vi "HFRR ADV v013 new software.vi"() -> ()   [LabVIEW 2025] (continued)
      event "Calibration": Value Change {
        n342 = event-data() -> ()  [unwired: 1 in, 6 out]
        n343 = local read "Calibration"() -> (w428:bool)
        n344 = case shown="False" w428 {
          frame False {
            n345 = property on="Calibration 2" class="TabCtl (strict)"("Visible"=FALSE) -> ()  [unwired: 2 in, 2 out]
            n346 = local write "Cal Password"("" ("Cal Password")) -> ()
          }
          frame True {
            n347 = property on="Calibration 2" class="TabCtl (strict)"("Visible"=TRUE) -> ()  [unwired: 2 in, 2 out]
            n348 = local write "Cal Password"("" ("Cal Password")) -> ()
          }
        }
        n349 = property on="Wrong Password" class="Str"("Visible"=FALSE) -> ()  [unwired: 2 in, 2 out]
      }
      event "Cal Password": Value Change {
        n350 = event-data() -> ()  [unwired: 1 in, 6 out]
        n351 = local read "Cal Password"() -> (w436:string)
        n352 = call <vilib>:"Trim Whitespace.vi"("string"=w436) -> ("trimmed string"=w435:string)  [unwired: 1 in]
        n353 = Equal?(x=w435, y="Cal@321") -> (x = y?=w433:bool)
        n354 = case shown="True" w433 {
          frame False {
            n355 = property on="Wrong Password" class="Str"("Visible"=TRUE) -> ()  [unwired: 2 in, 2 out]
          }
          frame True {
            n356 = property on="Wrong Password" class="Str"("Visible"=FALSE) -> ()  [unwired: 2 in, 2 out]
            n357 = local write "Main Tab"(T2."About" ("Main Tab")) -> ()
            n358 = local write "Cal Password"("" ("Cal Password")) -> ()
            n359 = local write "Main Dashboard Buttons"(T1."About" ("Main Dashboard Buttons")) -> ()
            n360 = local write "Tab Control 5"(T11."Temperature Calibration" ("Tab Control 5")) -> ()
            n361 = property on="Calibration 2" class="TabCtl (strict)"("Visible"=FALSE) -> ()  [unwired: 2 in, 2 out]
            n362 = property on="Tab Control 5" class="TabCtl (strict)"("Tabs Visible?"=FALSE ("Page Labels Display Visible?")) -> ()  [unwired: 2 in, 2 out]
            n363 = local write "Calibration"(FALSE ("Calibration")) -> ()
          }
        }
      }
      event "Calibration Selection": Value Change {
        n364 = event-data() -> ()  [unwired: 1 in, 6 out]
        n365 = local read "Calibration Selection"() -> (w447:T8)
        n366 = case shown="\"Stroke Calibration\"" w447 {
          tunnel: [T7."Stroke" ("Main Calibration Tab") T7."Friction" ("Main Calibration Tab") T7."Main" ("Main Calibration Tab") T7."Temperature" ("Main Calibration Tab")] -> w446
          frame "Stroke Calibration" {
          }
          frame "Friction Force Calibration" {
          }
          frame Default {
          }
          frame "Temperature Calibration" {
          }
        }
        n367 = local write "Main Calibration Tab"(w446) -> ()
      }
      event "Back Stroke": Value Change {
        n368 = event-data() -> ()  [unwired: 1 in, 6 out]
        n369 = local write "Main Stroke Tab"(T9."Step 1" ("Main Stroke Tab")) -> ()
        n370 = local write "Main Calibration Tab"(T7."Main" ("Main Calibration Tab")) -> ()
        n371 = local write "Back Stroke"(FALSE ("Back Stroke")) -> ()
      }
      event "Step 2 Back": Value Change {
        n372 = event-data() -> ()  [unwired: 1 in, 6 out]
        n373 = local write "Main Stroke Tab"(T9."Step 1" ("Main Stroke Tab")) -> ()
        n374 = local write "Step 2 Back"(FALSE ("Back Stroke")) -> ()
      }
      event "Step 3 Back": Value Change {
        n375 = event-data() -> ()  [unwired: 1 in, 6 out]
        n376 = local write "Main Stroke Tab"(T9."Step 2" ("Main Stroke Tab")) -> ()
        n377 = local write "Step 3 Back"(FALSE ("Back Stroke")) -> ()
      }
      event "Step 4 Back": Value Change {
        n378 = event-data() -> ()  [unwired: 1 in, 6 out]
        n379 = local write "Main Stroke Tab"(T9."Step 3" ("Main Stroke Tab")) -> ()
        n380 = local write "Step 4 Back"(FALSE ("Back Stroke")) -> ()
      }
      event "Step 5 Back": Value Change {
        n381 = event-data() -> ()  [unwired: 1 in, 6 out]
        n382 = local write "Main Stroke Tab"(T9."Step 4" ("Main Stroke Tab")) -> ()
        n383 = local write "Step 5 Back"(FALSE ("Back Stroke")) -> ()
      }
      event "Step 6 Back": Value Change {
        n384 = event-data() -> ()  [unwired: 1 in, 6 out]
        n385 = local write "Main Stroke Tab"(T9."Step 5" ("Main Stroke Tab")) -> ()
        n386 = local write "Step 6 Back"(FALSE ("Back Stroke")) -> ()
      }
      event "Back Stroke step 7": Value Change {
        n387 = event-data() -> ()  [unwired: 1 in, 6 out]
        n388 = local write "Main Stroke Tab"(T9."Step 6" ("Main Stroke Tab")) -> ()
        n389 = local write "Back Stroke step 7"(FALSE ("Back Stroke")) -> ()
      }
      event "Back Stroke step 8": Value Change {
        n390 = event-data() -> ()  [unwired: 1 in, 6 out]
        n391 = local write "Main Stroke Tab"(T9."Step 7" ("Main Stroke Tab")) -> ()
        n392 = local write "Back Stroke step 8"(FALSE ("Back Stroke")) -> ()
      }
      event "Back Stroke 8": Value Change {
        n393 = event-data() -> ()  [unwired: 1 in, 6 out]
        n394 = local write "MOVE CARRIAGE TO"(0.0 ("MOVE CARRIAGE TO")) -> ()
        n395 = local write "Main Stroke Tab"(T9."Step 1" ("Main Stroke Tab")) -> ()
        n396 = local write "Back Stroke 8"(FALSE ("Back Stroke 8")) -> ()
      }
      event "Continue Stroke": Value Change {
        n397 = event-data() -> ()  [unwired: 1 in, 6 out]
        n398 = local write "Main Stroke Tab"(T9."Step 2" ("Main Stroke Tab")) -> ()
        n399 = local write "Continue Stroke"(FALSE ("Continue Stroke")) -> ()
      }
      event "Continue Stroke step 2": Value Change {
        n400 = event-data() -> ()  [unwired: 1 in, 6 out]
        n401 = local write "Main Stroke Tab"(T9."Step 3" ("Main Stroke Tab")) -> ()
        n402 = local write "Continue Stroke step 2"(FALSE ("Continue Stroke")) -> ()
      }
      event "Continue Stroke step 3": Value Change {
        n403 = event-data() -> ()  [unwired: 1 in, 6 out]
        n404 = local write "Main Stroke Tab"(T9."Step 4" ("Main Stroke Tab")) -> ()
        n405 = local write "Continue Stroke step 3"(FALSE ("Continue Stroke")) -> ()
      }
      event "Continue Stroke step 4": Value Change {
        n406 = event-data() -> ()  [unwired: 1 in, 6 out]
        n407 = local write "Main Stroke Tab"(T9."Step 5" ("Main Stroke Tab")) -> ()
        n408 = local write "Continue Stroke step 4"(FALSE ("Continue Stroke")) -> ()
      }
      event "Continue Stroke step 5": Value Change {
        n409 = event-data() -> ()  [unwired: 1 in, 6 out]
        n410 = local write "Main Stroke Tab"(T9."Step 6" ("Main Stroke Tab")) -> ()
        n411 = local write "Continue Stroke step 5"(FALSE ("Continue Stroke")) -> ()
      }
      event "Continue Stroke step 6": Value Change {
        n412 = event-data() -> ()  [unwired: 1 in, 6 out]
        n413 = local write "Main Stroke Tab"(T9."Step 7" ("Main Stroke Tab")) -> ()
        n414 = local write "Continue Stroke step 6"(FALSE ("Continue Stroke")) -> ()
      }
      event "Continue Stroke step 7": Value Change {
        w485 = FALSE ("0.2mm")
        n415 = event-data() -> ()  [unwired: 1 in, 6 out]
        n416 = local write "0.4 mm"(w485) -> ()
        n417 = local write "0.6 mm"(w485) -> ()
        n418 = local write "1.0 mm"(w485) -> ()
        n419 = local write "1.2 mm"(w485) -> ()
        n420 = local write "0.2 2"(w485) -> ()
        n421 = local write "0.4 2"(w485) -> ()
        n422 = local write "0.6 2"(w485) -> ()
        n423 = local write "0.8 2"(w485) -> ()
        n424 = local write "1.0 2"(w485) -> ()
        n425 = local write "1.2"(w485) -> ()
        n426 = local write "0.2mm"(w485) -> ()
        n427 = local write "0.8mm"(w485) -> ()
        n428 = local write "Main Stroke Tab"(T9."Step 8" ("Main Stroke Tab")) -> ()
        n429 = local write "Continue Stroke step 7"(FALSE ("Continue Stroke")) -> ()
        n430 = local write "Stroke Test Complete"(T10."Test Progress" ("Stroke Test Complete")) -> ()
        "Position Measurment Temp" <- 0.0 ("Position Measurment Temp")
        "Calibration Tare" <- TRUE ("Calibration Tare")
      }
      event "Continue Stroke step 8": Value Change {
        n431 = event-data() -> ()  [unwired: 1 in, 6 out]
        n432 = local read "LVDT STROKE  Calibration"() -> (w490:dbl)
        n433 = local read "Position Measurment Temp"() -> (w491:dbl)
        n434 = case shown="7" w491 {
          selector: w491 -> [w496 w501 w506 w511 w516 w521 w524 w525]
          tunnel: w490 -> [w492 w497 w502 w507 w512 w517 _ _]
          frame 0, Default {
            w494 = TRUE ("0.2mm")
            n435 = Increment(x=w496) -> (x+1=w495:i32)
            n436 = local write "Position Measurment Temp"(w495) -> ()
            n437 = local write "0.2mm"(w494) -> ()
            n438 = local write "0.2 2"(w494) -> ()
            n439 = local write "MOVE CARRIAGE TO"(0.2 ("MOVE CARRIAGE TO")) -> ()
            "Calibration 0.2" <- w492
          }
          frame 1 {
            w499 = TRUE ("0.4 mm")
            n440 = Increment(x=w501) -> (x+1=w500:i32)
            n441 = local write "Calibration 0.4"(w497) -> ()
            n442 = local write "Position Measurment Temp"(w500) -> ()
            n443 = local write "0.4 mm"(w499) -> ()
            n444 = local write "MOVE CARRIAGE TO"(0.4 ("MOVE CARRIAGE TO")) -> ()
            n445 = local write "0.4 2"(w499) -> ()
          }
          frame 2 {
            w504 = TRUE ("0.6 mm")
            n446 = Increment(x=w506) -> (x+1=w505:i32)
            n447 = local write "Calibration 0.6"(w502) -> ()
            n448 = local write "Position Measurment Temp"(w505) -> ()
            n449 = local write "0.6 2"(w504) -> ()
            n450 = local write "0.6 mm"(w504) -> ()
            n451 = local write "MOVE CARRIAGE TO"(0.6 ("MOVE CARRIAGE TO")) -> ()
          }
          frame 3 {
            w508 = TRUE ("0.6 mm")
            n452 = Increment(x=w511) -> (x+1=w510:i32)
            n453 = local write "Position Measurment Temp"(w510) -> ()
            n454 = local write "MOVE CARRIAGE TO"(0.8 ("MOVE CARRIAGE TO")) -> ()
            n455 = local write "0.8mm"(w508) -> ()
            n456 = local write "0.8 2"(w508) -> ()
            "Calibration 0.8" <- w507
          }
          frame 4 {
            w513 = TRUE ("0.6 mm")
            n457 = Increment(x=w516) -> (x+1=w515:i32)
            n458 = local write "Position Measurment Temp"(w515) -> ()
            n459 = local write "MOVE CARRIAGE TO"(1.0 ("MOVE CARRIAGE TO")) -> ()
            n460 = local write "1.0 mm"(w513) -> ()
            n461 = local write "1.0 2"(w513) -> ()
            "Calibration 1.0" <- w512
          }
          frame 5 {
            w518 = TRUE ("0.6 mm")
            n462 = Increment(x=w521) -> (x+1=w520:i32)
            n463 = local write "Position Measurment Temp"(w520) -> ()
            n464 = local write "MOVE CARRIAGE TO"(1.2 ("MOVE CARRIAGE TO")) -> ()
            n465 = local write "1.2 mm"(w518) -> ()
            n466 = local write "1.2"(w518) -> ()
            "Calibration 1.2" <- w517
          }
          frame 6 {
            n467 = Increment(x=w524) -> (x+1=w523:i32)
            n468 = local write "Position Measurment Temp"(w523) -> ()
            n469 = local write "Stroke Test Complete"(T10."Stroke Points Completed" ("Stroke Test Complete")) -> ()
          }
          frame 7 {
            n470 = stacked-sequence {
              tunnel: w525 -> [w526 _ _]
              frame #0 {
                n471 = Increment(x=w526) -> (x+1=w527:i32)
                n472 = local write "Main Stroke Tab"(T9."Step 9" ("Main Stroke Tab")) -> ()
                n473 = local write "Position Measurment Temp"(w527) -> ()
                n474 = Insert Into Array(array=dbl[] [], new element #1=0.2 ("new element/subarray"), new element #2=0.4 ("new element/subarray"), new element #3=0.6 ("new element/subarray"), new element #4=0.8 ("new element/subarray"), new element #5=1.0 ("new element/subarray"), new element #6=1.2 ("new element/subarray")) -> (→"1D stroke":dbl[])  [unwired: 1 in]
                n475 = local read "Calibration 0.2"() -> (w534:dbl)
                n476 = local read "Calibration 0.4"() -> (w533:dbl)
                n477 = local read "Calibration 0.6"() -> (w532:dbl)
                n478 = local read "Calibration 0.8"() -> (w531:dbl)
                n479 = local read "Calibration 1.0"() -> (w530:dbl)
                n480 = local read "Calibration 1.2"() -> (w529:dbl)
                n481 = Insert Into Array(array=dbl[] [], new element #1=w534, new element #2=w533, new element #3=w532, new element #4=w531, new element #5=w530, new element #6=w529) -> (→"Calibrated Voltage Value":dbl[])  [unwired: 1 in]
              }
              frame #1 {
                n482 = local read "Calibrated Voltage Value"() -> (w546:dbl[])
                n483 = local read "1D stroke"() -> (w547:dbl[])
                n484 = for {
                  tunnel: [w550] -> w545 mode=indexing
                  tunnel: w547 -> [w549] mode=indexing
                  tunnel: w546 -> [w548] mode=indexing
                  n485 = formula code="if (stroke == 0.2) {\n    status = (voltage >= 0.0961 && voltage <= 0.4961) ? 1 : 0;\n} else if (stroke == 0.4) {\n    status = (voltage >= 0.3425 && voltage <= 0.7425) ? 1 : 0;\n} else if (stroke == 0.6) {\n    status = (voltage >= 0.5370 && voltage <= 0.9370) ? 1 : 0;\n} else if (stroke == 0.8) {\n    status = (voltage >= 0.6640 && voltage <= 1.0640) ? 1 : 0;\n} else if (stroke == 1.0) {\n    status = (voltage >= 0.9000 && voltage <= 1.1000) ? 1 : 0;\n} else if (stroke == 1.2) {\n    status = (voltage >= 0.9278 && voltage <= 1.3278) ? 1 : 0;\n} else {\n    status = 0; // Fails if an invalid stroke value is supplied\n}"("stroke"=w549, "voltage"=w548) -> ("status"=w550:dbl)
                }
                "Status" <- w545
              }
              frame #2 {
                w557 = 1.0
                n486 = local read "Status"() -> (w564:dbl[])
                n487 = Index Array(array=w564) -> (element #1=w563:dbl, element #2=w562:dbl, element #3=w561:dbl, element #4=w560:dbl, element #5=w559:dbl, element #6=w558:dbl)  [unwired: 6 in]
                n488 = Equal?(x=w562, y=w557) -> (x = y?=w555:bool)
                n489 = Equal?(x=w561, y=w557) -> (x = y?=w554:bool)
                n490 = Equal?(x=w560, y=w557) -> (x = y?=w553:bool)
                n491 = Equal?(x=w559, y=w557) -> (x = y?=w552:bool)
                n492 = Equal?(x=w558, y=w557) -> (x = y?=w551:bool)
                n493 = Equal?(x=w563, y=w557) -> (x = y?=w556:bool)
                n494 = case shown="True" w556 {
                  selector: w556 -> [w575 w576]
                  frame True {
                    n495 = local write "Point 1 - 0.2 mm"(w575) -> ()
                    n496 = property on="Point 1 - 0.2 mm" class="Bool"("Caption.Visible"=w575) -> ()  [unwired: 2 in, 2 out]
                  }
                  frame False {
                    n497 = local write "Point 1 - 0.2 mm"(w576) -> ()
                    n498 = property on="Point 1 - 0.2 mm" class="Bool"("Caption.Visible"=w576) -> ()  [unwired: 2 in, 2 out]
                  }
                }
                n499 = case shown="True" w555 {
                  selector: w555 -> [w573 w574]
                  frame True {
                    n500 = local write "Point 2 - 0.4 mm"(w573) -> ()
                    n501 = property on="Point 2 - 0.4 mm" class="Bool"("Caption.Visible"=w573) -> ()  [unwired: 2 in, 2 out]
                  }
                  frame False {
                    n502 = local write "Point 2 - 0.4 mm"(w574) -> ()
                    n503 = property on="Point 2 - 0.4 mm" class="Bool"("Caption.Visible"=w574) -> ()  [unwired: 2 in, 2 out]
                  }
                }
                n504 = case shown="True" w552 {
                  selector: w552 -> [w567 w568]
                  frame True {
                    n505 = local write "Point 5 - 1.0 mm"(w567) -> ()
                    n506 = property on="Point 5 - 1.0 mm" class="Bool"("Caption.Visible"=w567) -> ()  [unwired: 2 in, 2 out]
                  }
                  frame False {
                    n507 = local write "Point 5 - 1.0 mm"(w568) -> ()
                    n508 = property on="Point 5 - 1.0 mm" class="Bool"("Caption.Visible"=w568) -> ()  [unwired: 2 in, 2 out]
                  }
                }
                n509 = case shown="True" w554 {
                  selector: w554 -> [w571 w572]
                  frame True {
                    n510 = local write "Point 3 - 0.6 mm"(w571) -> ()
                    n511 = property on="Point 3 - 0.6 mm" class="Bool"("Caption.Visible"=w571) -> ()  [unwired: 2 in, 2 out]
                  }
                  frame False {
                    n512 = local write "Point 3 - 0.6 mm"(w572) -> ()
                    n513 = property on="Point 3 - 0.6 mm" class="Bool"("Caption.Visible"=w572) -> ()  [unwired: 2 in, 2 out]
                  }
                }
                n514 = case shown="True" w553 {
                  selector: w553 -> [w569 w570]
                  frame True {
                    n515 = local write "Point 4 - 0.8 mm"(w569) -> ()
                    n516 = property on="Point 4 - 0.8 mm" class="Bool"("Caption.Visible"=w569) -> ()  [unwired: 2 in, 2 out]
                  }
                  frame False {
                    n517 = local write "Point 4 - 0.8 mm"(w570) -> ()
                    n518 = property on="Point 4 - 0.8 mm" class="Bool"("Caption.Visible"=w570) -> ()  [unwired: 2 in, 2 out]
                  }
                }
                n519 = case shown="True" w551 {
                  selector: w551 -> [w565 w566]
                  frame True {
                    n520 = local write "Point 6 - 1.2 mm"(w565) -> ()
                    n521 = property on="Point 6 - 1.2 mm" class="Bool"("Caption.Visible"=w565) -> ()  [unwired: 2 in, 2 out]
                  }
                  frame False {
                    n522 = local write "Point 6 - 1.2 mm"(w566) -> ()
                    n523 = property on="Point 6 - 1.2 mm" class="Bool"("Caption.Visible"=w566) -> ()  [unwired: 2 in, 2 out]
                  }
                }
              }
            }
          }
        }
      }
      event "Quit": Value Change {
        n524 = event-data() -> ()  [unwired: 1 in, 6 out]
      }
    }
    n525 = Wait (ms)(milliseconds to wait=u32 100) -> ()  [unwired: 1 out]
  }
  n526 = while {
    stop <- w579 stop-if-true
    n527 = Wait (ms)(milliseconds to wait=u32 200) -> ()  [unwired: 1 out]
    n528 = local read "Quit"() -> (w579:bool)
  }
  n529 = while {
    shift-right: [w581] -> _
    shift-left: "Enum - Selector" -> [w582]
    stop <- w583 stop-if-true
    # "Auto Start Logic Loop"
    n530 = case shown="\"Maintain Stage\"" w582 {
      tunnel: [w586 w592 w619 w651 w681 Auto_Start_enum."Exit" ("Enum - Selector") Auto_Start_enum."Init" ("Enum - Selector")] -> w581
      frame "Init", Default {
        n531 = local read "Auto Start Test"() -> (w585:bool)
        n532 = Select(t=Auto_Start_enum."Humidity & Temperature On" ("Enum - Selector"), s=w585, f=Auto_Start_enum."Init") -> (s? t:f=w586:T14)
      }
      frame "Humidity & Temperature On" {
        n533 = stacked-sequence {
          tunnel: [_ _ _ _ _ _ Auto_Start_enum."Reach point" ("Enum - Selector")] -> w589
          frame #0 {
            w594 = T17."Disabled and Grayed Out" ("Disabled")
            w595 = TRUE ("Heater Button")
            n534 = property on="Humidity" class="Bool (strict)"("DisabledEnum"=w594) -> ()  [unwired: 2 in, 2 out]
            n535 = property on="Heater Button" class="Bool (strict)"("DisabledEnum"=w594) -> ()  [unwired: 2 in, 2 out]
            n536 = local write "Heater Button"(w595) -> ()
            n537 = local write "Humidity"(w595) -> ()
            n538 = property on="Heater Button" class="Bool (strict)"("Val(Sgnl)"=TRUE ("Value (Signaling)")) -> ()  [unwired: 2 in, 2 out]
          }
          frame #1 {
            n539 = Wait (ms)(milliseconds to wait=u32 3000) -> ()  [unwired: 1 out]
          }
          frame #2 {
            n540 = local read "Set Temp"() -> (w601:dbl)
            n541 = Number To Fractional String(number=w601, precision (6)=i16 2) -> (F-format string=w598:string)  [unwired: 2 in]
            n542 = Concatenate Strings("ST;" ("Command"), w598) -> (w599:string)
            n543 = local write "Command"(w599) -> ()
          }
          frame #3 {
            n544 = Wait (ms)(milliseconds to wait=u32 1500) -> ()  [unwired: 1 out]
          }
          frame #4 {
            (unwired) i16 2 ("precision (6)")
            n545 = local read "Set Rh"() -> (w604:dbl)
            n546 = Number To Fractional String(number=w604) -> (F-format string=w607:string)  [unwired: 3 in]
            n547 = local read "WriteHumidity"() -> (w605:string[])
            n548 = Concatenate Strings("M;" ("new element/subarray"), w607) -> (w608:string)
            n549 = local write "Command"("HE;1" ("Command")) -> ()
            n550 = Insert Into Array(array=w605, new element=w608) -> (w606:string[])  [unwired: 1 in]
            n551 = local write "WriteHumidity"(w606) -> ()
          }
          frame #5 {
            n552 = Wait (ms)(milliseconds to wait=u32 1500) -> ()  [unwired: 1 out]
          }
          frame #6 {
            w611 = TRUE ("Reach point temp")
            n553 = local write "Reach point Humidity"(w611) -> ()
            n554 = local write "Reach point temp"(w611) -> ()
          }
        }
        n555 = local read "Auto Start Test"() -> (w591:bool)
        n556 = Not(x=w591) -> (.not. x?=w590:bool)
        n557 = Select(t=Auto_Start_enum."close", s=w590, f=w589) -> (s? t:f=w592:T14)
      }
      frame "Reach point" {
        w620 = TRUE ("PAUSE")
        w628 = 1.0 ("y")
        w631 = 1.0 ("y")
        n558 = local read "Set Temp"() -> (w613:dbl)
        n559 = local read "Set Humidity:"() -> (w627:dbl)
        n560 = local read "Humidity ( %RH )"() -> (w632:dbl)
        n561 = Add(x=w613, y=w631) -> (x+y=w630:dbl)
        n562 = Subtract(x=w613, y=w631) -> (x-y=w629:dbl)
        n563 = Add(x=w627, y=w628) -> (x+y=w626:dbl)
        n564 = Subtract(x=w627, y=w628) -> (x-y=w625:dbl)
        n565 = local read "TEMP"() -> (w633:dbl)
        n566 = In Range and Coerce(upper limit=w626, x=w632, lower limit=w625) -> (In Range?=w614:bool)  [unwired: 1 out]
        n567 = In Range and Coerce(upper limit=w630, x=w633, lower limit=w629) -> (In Range?=w615:bool)  [unwired: 1 out]
        n568 = case shown="True" w614 {
          frame False {
          }
          frame True {
            n569 = case shown="True" "Reach point Humidity" {
              selector: "Reach point Humidity" -> [_ w639]
              frame False {
              }
              frame True {
                n570 = local read "EVENT LOG"() -> (w636:string)
                n571 = Not(x=w639) -> (.not. x?=w638:bool)
                n572 = local write "Reach point Humidity"(w638) -> ()
                n573 = call "Event Log.vi"("Content"="Target Humidity reached", "EVENT LOG"=w636) -> ("EVENT LOG"=w637:string)  [unwired: 8 in, 1 out]
                n574 = local write "EVENT LOG"(w637) -> ()
              }
            }
          }
        }
        n575 = case shown="True" w615 {
          frame False {
          }
          frame True {
            n576 = case shown="True" "Reach point temp" {
              selector: "Reach point temp" -> [_ w645]
              frame False {
              }
              frame True {
                n577 = local read "EVENT LOG"() -> (w642:string)
                n578 = Not(x=w645) -> (.not. x?=w644:bool)
                n579 = local write "Reach point temp"(w644) -> ()
                n580 = call "Event Log.vi"("Content"="Target Temperature reached", "EVENT LOG"=w642) -> ("EVENT LOG"=w643:string)  [unwired: 8 in, 1 out]
                n581 = local write "EVENT LOG"(w643) -> ()
              }
            }
          }
        }
        n582 = local read "Auto Start Test"() -> (w618:bool)
        n583 = And(x=w615, y=w614) -> (x .and. y?=w624:bool)
        n584 = Select(t=Auto_Start_enum."Maintain Stage" ("Enum - Selector"), s=w624, f=Auto_Start_enum."Reach point" ("Enum - Selector")) -> (s? t:f=w621:T14)
        n585 = Not(x=w618) -> (.not. x?=w617:bool)
        n586 = Select(t=Auto_Start_enum."close", s=w617, f=w621) -> (s? t:f=w619:T14)
        n587 = call "ELAPSED TIMER VI.vi"("RESET"=w620, "PAUSE"=w620) -> ()  [unwired: 7 in, 3 out]
      }
      frame "Maintain Stage" {
        w660 = 2.0 ("y")
        w659 = 1.0 ("y")
        # "Humidity and  temperatures Set Point  have been reached"
        n588 = local read "Set Temp"() -> (w646:dbl)
        n589 = local read "Set Humidity:"() -> (w663:dbl)
        n590 = local read "Humidity ( %RH )"() -> (w666:dbl)
        n591 = Add(x=w646, y=w659) -> (x+y=w665:dbl)
        n592 = Subtract(x=w646, y=w659) -> (x-y=w664:dbl)
        n593 = local read "TEMP"() -> (w667:dbl)
        n594 = Add(x=w663, y=w660) -> (x+y=w662:dbl)
        n595 = Subtract(x=w663, y=w660) -> (x-y=w661:dbl)
        n596 = In Range and Coerce(upper limit=w665, x=w667, lower limit=w664) -> (In Range?=w658:bool)  [unwired: 1 out]
        n597 = In Range and Coerce(upper limit=w662, x=w666, lower limit=w661) -> (In Range?=w657:bool)  [unwired: 1 out]
        n598 = And(x=w658, y=w657) -> (x .and. y?=w656:bool)
        n599 = Not(x=w656) -> (.not. x?=w655:bool)
        n600 = call "ELAPSED TIMER VI.vi"("TARGET"=60.0, "RESET"=w655, "PAUSE"=FALSE) -> ("ELAPSED INDICATION"=w652:bool)  [unwired: 6 in, 2 out]
        n601 = case shown="True" w652 {
          tunnel: w652 -> [_ w670]
          tunnel: [Auto_Start_enum."Maintain Stage" ("Enum - Selector") w669] -> w650
          frame False {
          }
          frame True {
            n602 = stacked-sequence {
              tunnel: w670 -> [_ _ _ _ _]
              tunnel: [_ _ _ _ Auto_Start_enum."Start Stage" ("Enum - Selector")] -> w669
              frame #0 {
                n603 = local read "EVENT LOG"() -> (w672:string)
                n604 = call "Event Log.vi"("Content"="Humidity and temperature set point has stabilized.", "EVENT LOG"=w672) -> ("EVENT LOG"=w673:string)  [unwired: 8 in, 1 out]
                n605 = local write "EVENT LOG"(w673) -> ()
              }
              frame #1 {
                n606 = Wait (ms)(milliseconds to wait=u32 100) -> ()  [unwired: 1 out]
              }
              frame #2 {
                n607 = local read "EVENT LOG"() -> (w676:string)
                n608 = call "Event Log.vi"("Content"="Auto Test Started", "EVENT LOG"=w676) -> ("EVENT LOG"=w677:string)  [unwired: 8 in, 1 out]
                n609 = local write "EVENT LOG"(w677) -> ()
              }
              frame #3 {
                w678 = TRUE ("RUN")
                n610 = local write "RUN"(w678) -> ()
                n611 = property on="Auto Start Temp" class="Bool (strict)"("Val(Sgnl)"=w678) -> ()  [unwired: 2 in, 2 out]
                "Auto Start Temp" <- w678
              }
              frame #4 {
              }
            }
          }
        }
        n612 = local read "Auto Start Test"() -> (w649:bool)
        n613 = Not(x=w649) -> (.not. x?=w648:bool)
        n614 = Select(t=Auto_Start_enum."close", s=w648, f=w650) -> (s? t:f=w651:T14)
      }
      frame "Start Stage" {
        w680 = TRUE ("PAUSE")
        n615 = local read "Auto Start Test"() -> (w685:bool)
        n616 = Not(x=w685) -> (.not. x?=w684:bool)
        n617 = Select(t=Auto_Start_enum."close" ("Enum - Selector"), s=w684, f=Auto_Start_enum."Start Stage" ("Enum - Selector")) -> (s? t:f=w681:T14)
        n618 = call "ELAPSED TIMER VI.vi"("RESET"=w680, "PAUSE"=w680) -> ()  [unwired: 7 in, 3 out]
      }
      frame "close" {
        w687 = FALSE ("Heater Button")
        n619 = local write "RUN"(w687) -> ()
        n620 = local write "Heater Button"(w687) -> ()
        n621 = local write "Humidity"(w687) -> ()
        n622 = local write "Auto Start Test"(w687) -> ()
        n623 = property on="Heater Button" class="Bool (strict)"("Val(Sgnl)"=FALSE ("Value (Signaling)")) -> ()  [unwired: 2 in, 2 out]
      }
      frame "Exit" {
      }
    }
    n624 = Wait (ms)(milliseconds to wait=u32 100) -> ()  [unwired: 1 out]
    n625 = local read "Quit"() -> (w583:bool)
  }
  n626 = property on="Service Password Log" class="Str"("Visible"=w14) -> ()  [unwired: 2 in, 2 out]
  n627 = property on="Password 3" class="Clust (strict)"("Visible"=w14) -> ()  [unwired: 2 in, 2 out]
  n628 = while {
    stop <- w716 stop-if-true
    w699 = errorcluster {"status"=FALSE, "code"=0, "source"=""} ("error in (no error) 3")
    # "this loop is for manual report generation"
    n629 = local read "Confirm Measrurement"() -> (w698:bool)
    n630 = case shown="True" w698 {
      selector: w698 -> [_ w806]
      tunnel: errorcluster {"status"=FALSE, "code"=0, "source"=""} ("error in (no error) 3") -> [_ w807]
      tunnel: [_ w805] -> _
      frame False {
      }
      frame True {
        n631 = stacked-sequence {
          tunnel: w807 -> [_ w840 _]
          tunnel: w806 -> [_ _ w947]
          tunnel: [_ w828 _] -> w805
          frame #0 {
            n632 = String To Path(string="C:\\LAB-IQ\\Image Calibrate v01.dcf") -> (path=w810:path)
            n633 = Open/Create/Replace File ("Open File")(file path (use dialog)=w810) -> (refnum out=w811:refnum<file>)  [unwired: 5 in, 2 out]
            n634 = for {
              N: 4 -> [_]
              tunnel: w811 -> [w817]
              i -> [w813]
              n635 = Read from Text File ("Read File")(file (use dialog)=w817) -> (text=w818:string)  [unwired: 3 in, 3 out]
              n636 = String Subset(string=w818, offset (0)=6, length (rest)=10 ("length (rest)")) -> (substring=w814:string)
              n637 = Fract/Exp String To Number(string=w814) -> (number=w812:dbl)  [unwired: 3 in, 1 out]
              n638 = case shown="3" w813 {
                tunnel: w812 -> [w819 w820 _ w821 _]
                frame 0 {
                  n639 = local write "5x Gain"(w819) -> ()
                }
                frame 1 {
                  n640 = local write "10x Gain"(w820) -> ()
                }
                frame 2 {
                }
                frame 3 {
                  n641 = local write "100x gain"(w821) -> ()
                }
                frame 4, Default {
                }
              }
            }
          }
          frame #1 {
            n642 = local read "TEST STANDARD"() -> (w823:T3)
            n643 = case shown="\"ISO 12156\"" w823 {
              tunnel: ["ASTM D6079" "ISO 12156"] -> w822
              frame "ASTM D6079", Default {
              }
              frame "ISO 12156" {
              }
            }
            n644 = call "IMAGE ANALYSIS.vi"("Enum"=POST_ANALYSIS_ENUM."GET MEASUREMENTS", "error in"=w840) -> ("error out"=w847:errorcluster)  [unwired: 8 in, 1 out]
            n645 = local read "Magnification :"() -> (w833:string)
            n646 = call "Stall Data Flow.vim"("value in"=w847, "milliseconds to wait"=u32 1000) -> ("value out"=w846:errorcluster)  [unwired: 1 out]
            n647 = local read "Test File List :"() -> (w844:string)
            n648 = case shown="\"10x\"" w833 {
              tunnel: [w883 w884] -> w831
              frame "5x", Default {
                n649 = local read "5x Gain"() -> (w883:dbl)
              }
              frame "10x" {
                # "5x"
                n650 = local read "10x Gain"() -> (w884:dbl)
              }
            }
            n651 = call "IMAGE ANALYSIS.vi"("Enum"=POST_ANALYSIS_ENUM."READ", "error in"=w846) -> ("error out"=w843:errorcluster, "data out"=w834:string)  [unwired: 8 in]
            n652 = Match Pattern(string=w834, regular expression="\"type\": ") -> (after substring=w838:string)  [unwired: 1 in, 3 out]
            n653 = call "IMAGE PATH CREATION PY.vi"("error in (no error)"=w843, "File Name :"=w844) -> ("error out"=w842:errorcluster, "File Path"=w830:path, "File Path String:"=w825:string)  [unwired: 7 in]
            n654 = Match Pattern(string=w838, regular expression=",") -> (before substring=w824:string)  [unwired: 1 in, 3 out]
            n655 = local read "Calibration Tab"() -> (w827:enum32{"Measrument", "Calibrate"})
            n656 = call "Stall Data Flow.vim"("value in"=w842, "milliseconds to wait"=u32 250) -> ("value out"=w826:errorcluster)  [unwired: 1 out]
            n657 = Equal?(x=w824, y="\"rectangle\"") -> (x = y?=w835:bool)
            n658 = case shown="False" w835 {
              tunnel: w834 -> [w889 w944]
              tunnel: w831 -> [_ w935]
              tunnel: cluster{"major":dbl, "minor":dbl, "average":dbl} {"major"=0.0, "minor"=0.0, "average"=0.0} -> [w887 w931]
              tunnel: [w886 w928] -> w829
              tunnel: w824 -> [w888 _]
              tunnel: w831 -> [w885 _]
              frame False {
                n659 = Equal?(x=w888, y="\"line\"") -> (x = y?=w890:bool)
                n660 = case shown="True" w890 {
                  tunnel: w889 -> [_ w905]
                  tunnel: w887 -> [w892 w904]
                  tunnel: [w892 w902] -> w886
                  tunnel: w885 -> [_ w901]
                  frame False {
                  }
                  frame True {
                    w900 = 0.0 ("Major Axis")
                    n661 = Match Pattern(string=w905, regular expression="\"length_px\":") -> (after substring=w903:string)  [unwired: 1 in, 3 out]
                    n662 = property on="Major Axis" class="DigNum (strict)"("Caption.Text"="") -> ()  [unwired: 2 in, 2 out]
                    n663 = property on="Minor Axis" class="DigNum (strict)"("Caption.Text"="") -> ()  [unwired: 2 in, 2 out]
                    n664 = property on="Average" class="DigNum (strict)"("Caption.Text"="Line") -> ()  [unwired: 2 in, 2 out]
                    n665 = Fract/Exp String To Number(string=w903, default (0 dbl)=0.0 ("default (0 DBL)")) -> (number=w899:dbl)  [unwired: 2 in, 1 out]
                    "Pixel Value" <- w899
                    n666 = Multiply(x=w899, y=w901) -> (x*y=w912:dbl)
                    n667 = Multiply(x=w912, y=1000.0) -> (x*y=w895:dbl)
                    n668 = Divide(x=w895, y=1000.0) -> (x/y=w898:dbl)
                    n669 = local write "Measurment (mm)"(w898) -> ()
                    n670 = Bundle By Name(cluster=w904, "average"=w895) -> (w902:cluster{"major":dbl, "minor":dbl, "average":dbl})
                    n671 = Number To Fractional String(number=w895, precision (6)=i16 1) -> (F-format string=w894:string)  [unwired: 2 in]
                    n672 = local write "Minor Axis"(w900) -> ()
                    n673 = local write "Major Axis"(w900) -> ()
                    n674 = Fract/Exp String To Number(string=w894) -> (number=w893:dbl)  [unwired: 3 in, 1 out]
                    n675 = local write "Average"(w893) -> ()
                  }
                }
              }
              frame True {
                w932 = 1000.0 ("y")
                w938 = 0.0 ("default (0 DBL)")
                n676 = Match Pattern(string=w944, regular expression=" \"width_px\":") -> (after substring=w942:string)  [unwired: 1 in, 3 out]
                n677 = Match Pattern(string=w942, regular expression="\"height_px\":") -> (before substring=w940:string, after substring=w939:string)  [unwired: 1 in, 2 out]
                n678 = Fract/Exp String To Number(string=w940, default (0 dbl)=w938) -> (number=w937:dbl)  [unwired: 2 in, 1 out]
                n679 = Fract/Exp String To Number(string=w939, default (0 dbl)=w938) -> (number=w936:dbl)  [unwired: 2 in, 1 out]
                n680 = Multiply(x=w937, y=w935) -> (x*y=w934:dbl)
                n681 = Multiply(x=w936, y=w935) -> (x*y=w933:dbl)
                n682 = Multiply(x=w934, y=w932) -> (x*y=w918:dbl)
                n683 = Multiply(x=w933, y=w932) -> (x*y=w916:dbl)
                n684 = Add(x=w918, y=w916) -> (x+y=w930:dbl)
                n685 = property on="Major Axis" class="DigNum (strict)"("Caption.Text"="Major Axis") -> ()  [unwired: 2 in, 2 out]
                n686 = property on="Minor Axis" class="DigNum (strict)"("Caption.Text"="Minor Axis") -> ()  [unwired: 2 in, 2 out]
                n687 = property on="Average" class="DigNum (strict)"("Caption.Text"="Average") -> ()  [unwired: 2 in, 2 out]
                n688 = Divide(x=w930, y=2.0) -> (x/y=w914:dbl)
                n689 = Bundle By Name(cluster=w931, "major"=w918, "minor"=w916, "average"=w914) -> (w928:cluster{"major":dbl, "minor":dbl, "average":dbl})
                n690 = Number To Fractional String(number=w916, precision (6)=i16 1) -> (F-format string=w923:string)  [unwired: 2 in]
                n691 = Number To Fractional String(number=w914, precision (6)=i16 1) -> (F-format string=w924:string)  [unwired: 2 in]
                n692 = Number To Fractional String(number=w918, precision (6)=i16 1) -> (F-format string=w922:string)  [unwired: 2 in]
                n693 = Fract/Exp String To Number(string=w923) -> (number=w915:dbl)  [unwired: 3 in, 1 out]
                n694 = Fract/Exp String To Number(string=w924) -> (number=w913:dbl)  [unwired: 3 in, 1 out]
                n695 = Fract/Exp String To Number(string=w922) -> (number=w917:dbl)  [unwired: 3 in, 1 out]
                n696 = local write "Major Axis"(w917) -> ()
                n697 = local write "Average"(w913) -> ()
                n698 = local write "Minor Axis"(w915) -> ()
              }
            }
            n699 = case shown="\"Measrument\", Default" w827 {
              tunnel: w830 -> [w857 _]
              tunnel: w829 -> [w856 _]
              tunnel: [w853 w882] -> w828
              tunnel: w826 -> [w855 w882]
              tunnel: w825 -> [w854 _]
              tunnel: w822 -> [w852 _]
              frame "Measrument", Default {
                n700 = stacked-sequence {
                  tunnel: w857 -> [w875 _]
                  tunnel: w856 -> [w873 _]
                  tunnel: w855 -> [w871 _]
                  tunnel: w854 -> [w870 _]
                  tunnel: [w865 _] -> w853
                  tunnel: w852 -> [w858 _]
                  frame #0 {
                    n701 = call "IMAGE ANALYSIS.vi"("Enum"=POST_ANALYSIS_ENUM."SAVE IMAGE", "error in"=w871, "IMAGE FILE PATH"=w870) -> ("error out"=w869:errorcluster)  [unwired: 7 in, 1 out]
                    n702 = call "Stall Data Flow.vim"("value in"=w869, "milliseconds to wait"=u32 1000) -> ("value out"=w860:errorcluster)  [unwired: 1 out]
                    n703 = local read "Test File List :"() -> (w877:string)
                    n704 = call "IMAGE ANALYSIS.vi"("Enum"=POST_ANALYSIS_ENUM."MINIMIZE UI", "error in"=w860) -> ("error out"=w867:errorcluster)  [unwired: 8 in, 1 out]
                    n705 = Bundle By Name(cluster=T24 {"File Name"="", "Test Method"="", "Operator"="", "Fuel Description"="", "Date and time"=""} ("Main Ref"), "Test Method"=w858, "File Name"=w877) -> (w878:T24)
                    n706 = call "Stall Data Flow.vim"("value in"=w867, "milliseconds to wait"=u32 1500) -> ("value out"=w862:errorcluster)  [unwired: 1 out]
                    n707 = call "duf file read.vi"("error in (no error)"=w862, "Main Ref"=w878) -> ("error out"=w876:errorcluster, "Main Ref 2"=w874:T24)  [unwired: 8 in]
                    n708 = call "DETECTION REPORT for manual.vi"("error in (no error)"=w876, "return value 3"=w873, "Image File Path"=w875, "Main Ref"=w874) -> ("error out"=w872:errorcluster)  [unwired: 7 in]
                    n709 = call <vilib>:"Clear Errors.vi"("error in (no error)"=w872) -> ("error out"=w863:errorcluster)  [unwired: 5 in, 1 out]
                    n710 = call "IMAGE ANALYSIS.vi"("Enum"=POST_ANALYSIS_ENUM."MINIMIZE UI", "error in"=w863) -> ("error out"=w865:errorcluster)  [unwired: 8 in, 1 out]
                  }
                  frame #1 {
                    n711 = local write "Main Tab"(T2."HOME" ("Main Tab")) -> ()
                    n712 = local write "Main Dashboard Buttons"(T1."Home" ("Main Dashboard Buttons")) -> ()
                  }
                }
              }
              frame "Calibrate" {
              }
            }
          }
          frame #2 {
            n713 = Not(x=w947) -> (.not. x?=w946:bool)
            n714 = local write "Confirm Measrurement"(w946) -> ()
            n715 = local read "Calibration Tab"() -> (w945:enum32{"Measrument", "Calibrate"})
            n716 = case shown="\"Measrument\", Default" w945 {
              frame "Measrument", Default {
                (unwired) T19."HOME" ("Main Tab")
                n717 = local write "Main Tab"(T2."HOME" ("Main Tab")) -> ()
              }
              frame "Calibrate" {
              }
            }
          }
        }
      }
    }
    n718 = local read "Humidity"() -> (w690:bool)
    n719 = local read "Save Change"() -> (w695:bool)
    n720 = local read "Calibrate"() -> (w696:bool)
    n721 = local read "Auto Start Test"() -> (w691:bool)
    n722 = case shown="True" w696 {
      selector: w696 -> [_ w803]
      frame False {
      }
      frame True {
        n723 = Not(x=w803) -> (.not. x?=w802:bool)
        n724 = local write "Calibrate"(w802) -> ()
        n725 = local write "Calibration Tab"(enum32{"Measrument", "Calibrate"}."Calibrate" ("Calibration Tab")) -> ()
      }
    }
    n726 = case shown="True" w695 {
      selector: w695 -> [_ w747]
      frame False {
      }
      frame True {
        n727 = stacked-sequence {
          tunnel: w747 -> [_ _ _ _ w801]
          frame #0 {
            n728 = call "IMAGE ANALYSIS.vi"("Enum"=POST_ANALYSIS_ENUM."HIDE UI") -> ()  [unwired: 9 in, 2 out]
          }
          frame #1 {
            n729 = local read "100x gain"() -> (w749:dbl)
            n730 = local read "10x Gain"() -> (w750:dbl)
            n731 = local read "5x Gain"() -> (w751:dbl)
            n732 = Number To Fractional String(number=w750, width (-)=i16 4, precision (6)=i16 7) -> (F-format string=w772:string)  [unwired: 1 in]
            n733 = Number To Fractional String(number=0.0, width (-)=i16 4, precision (6)=i16 7) -> (F-format string=w767:string)  [unwired: 1 in]
            n734 = Number To Fractional String(number=w749, width (-)=i16 4, precision (6)=i16 7) -> (F-format string=w755:string)  [unwired: 1 in]
            n735 = Number To Fractional String(number=w751, width (-)=i16 10 ("precision (6)"), precision (6)=i16 7) -> (F-format string=w781:string)  [unwired: 1 in]
            n736 = Concatenate Strings("[CH1]" ("string"), w781, " - 5x Gain" ("string"), "\r") -> (w771:string)
            n737 = Concatenate Strings("[CH2]" ("string"), w772, " - 10x Gain" ("string"), "\r") -> (w770:string)
            n738 = Concatenate Strings("[CH3]" ("string"), w767, " - 20x Gain" ("string"), "\r") -> (w761:string)
            n739 = Concatenate Strings("[CH4]" ("string"), w755, " - 100x Gain" ("string"), "\r") -> (w754:string)
            n740 = String To Path(string="C:\\LAB-IQ\\Image Calibrate v01.dcf") -> (path=w784:path)
            n741 = Concatenate Strings(w771, w770, w761, w754) -> (w769:string)
            n742 = call <vilib>:"Write Characters To File.vi"("append to file? (new file:F)"=FALSE, "character string"=w769, "file path (dialog if empty)"=w784) -> ()  [unwired: 2 in, 1 out]
          }
          frame #2 {
            n743 = String To Path(string="C:\\LAB-IQ\\Image Calibrate v01.dcf") -> (path=w787:path)
            n744 = Open/Create/Replace File ("Open File")(file path (use dialog)=w787) -> (refnum out=w788:refnum<file>)  [unwired: 5 in, 2 out]
            n745 = for {
              N: 4 -> [_]
              tunnel: w788 -> [w794]
              i -> [w790]
              n746 = Read from Text File ("Read File")(file (use dialog)=w794) -> (text=w795:string)  [unwired: 3 in, 3 out]
              n747 = String Subset(string=w795, offset (0)=6, length (rest)=10 ("length (rest)")) -> (substring=w791:string)
              n748 = Fract/Exp String To Number(string=w791) -> (number=w789:dbl)  [unwired: 3 in, 1 out]
              n749 = case shown="3" w790 {
                tunnel: w789 -> [w796 w797 _ w798 _]
                frame 0 {
                  n750 = local write "5x Gain"(w796) -> ()
                }
                frame 1 {
                  n751 = local write "10x Gain"(w797) -> ()
                }
                frame 2 {
                }
                frame 3 {
                  n752 = local write "100x gain"(w798) -> ()
                }
                frame 4, Default {
                }
              }
            }
          }
          frame #3 {
            n753 = call "IMAGE ANALYSIS.vi"("Enum"=POST_ANALYSIS_ENUM."SHOW UI") -> ()  [unwired: 9 in, 2 out]
          }
          frame #4 {
            n754 = Not(x=w801) -> (.not. x?=w800:bool)
            n755 = local write "Save Change"(w800) -> ()
          }
        }
      }
    }
    n756 = case shown="False" w691 {
      tunnel: w690 -> [w717 _]
      frame False {
        n757 = case shown="True" w717 {
          frame False {
          }
          frame True {
            n758 = local read "Set Humidity:"() -> (w721:dbl)
            n759 = local read "Set Humidity:"() -> (w724:dbl)
            n760 = local read "Humidity ( %RH )"() -> (w725:dbl)
            n761 = Subtract(x=w721, y=2.0) -> (x-y=w719:dbl)
            n762 = Add(x=w724, y=2.0) -> (x+y=w720:dbl)
            n763 = In Range and Coerce(upper limit=w720, x=w725, lower limit=w719) -> (In Range?=w718:bool)  [unwired: 1 out]
            n764 = case shown="True" w718 {
              frame False {
              }
              frame True {
                n765 = case shown="True" "Manual Humididty Reached" {
                  selector: "Manual Humididty Reached" -> [_ w728]
                  frame False {
                  }
                  frame True {
                    n766 = Not(x=w728) -> (.not. x?=w727:bool)
                    n767 = local write "Manual Humididty Reached"(w727) -> ()
                    n768 = local read "EVENT LOG"() -> (w730:string)
                    n769 = call "Event Log.vi"("Content"="Target Humidity reached", "EVENT LOG"=w730) -> ("EVENT LOG"=w729:string)  [unwired: 8 in, 1 out]
                    n770 = local write "EVENT LOG"(w729) -> ()
                  }
                }
              }
            }
          }
        }
      }
      frame True {
        n771 = local write "Manual Humididty Reached"(TRUE ("Manual Humididty Reached")) -> ()
      }
    }
    n772 = local read "Cap Live Image"() -> (w711:bool)
    n773 = local read "SCAR MEASURMENT"() -> (w714:enum32{"Auto Scar", "Manual Scar"})
    n774 = Wait (ms)(milliseconds to wait=u32 250) -> ()  [unwired: 1 out]
    n775 = Equal?(x=w714, y=enum32{"Auto Scar", "Manual Scar"}."Manual Scar" ("SCAR MEASURMENT")) -> (x = y?=w712:bool)
    n776 = And(x=w712, y=w711) -> (x .and. y?=w710:bool)
    n777 = case shown="True" w710 {
      selector: w710 -> [_ w1026]
      frame False {
      }
      frame True {
        n778 = stacked-sequence {
          tunnel: [_ _ _ w1041 _] -> _
          tunnel: w1026 -> [_ _ _ _ w1048]
          frame #0 {
            w1027 = 0.0
            n779 = local write "Major Axis"(w1027) -> ()
            n780 = local write "Minor Axis"(w1027) -> ()
            n781 = local write "Average"(w1027) -> ()
          }
          frame #1 {
            n782 = call "CAMERA LIVE FEED FGV.vi"("Enum - Menu"=CAMERA_LIVE_FEED_ENUM."CAMERA MINIMIZE") -> ()  [unwired: 9 in, 2 out]
          }
          frame #2 {
            n783 = local read "FILE 3"() -> (w1035:string)
            n784 = call <vilib>:"Trim Whitespace.vi"("string"="C:\\LAB-IQ\\images\\") -> ("trimmed string"=w1037:string)  [unwired: 1 in]
            n785 = String To Path(string=w1037) -> (path=w1036:path)
            n786 = Concatenate Strings(w1035, ".png" ("string")) -> (w1034:string)
            n787 = Build Path(base path=w1036, name or relative path=w1034) -> (appended path=w1032:path)
            n788 = Path To String(path=w1032) -> (string=w1031:string)
            n789 = call "CAMERA LIVE FEED FGV.vi"("Enum - Menu"=CAMERA_LIVE_FEED_ENUM."CAMERA SAVE", "Image Path"=w1031) -> ("error out"=w1029:errorcluster)  [unwired: 8 in, 1 out]
            n790 = case shown="No Error" w1029 {
              frame No Error {
                n791 = One Button Dialog(message="Image saved successfully") -> ()  [unwired: 1 in, 1 out]
              }
              frame Error {
              }
            }
          }
          frame #3 {
            n792 = call "LIST FILE NAMES.vi"() -> ("error out"=w1043:errorcluster, "filenames"=w1040:string[])  [unwired: 10 in]
            n793 = call "IMAGE ANALYSIS.vi"("Enum"=POST_ANALYSIS_ENUM."SHOW UI", "error in"=w1043) -> ("error out"=w1041:errorcluster)  [unwired: 8 in, 1 out]
            n794 = property on="Test File List :" class="CmbBox"("Strings[]"=w1040) -> ()  [unwired: 2 in, 2 out]
          }
          frame #4 {
            (unwired) T23."Report" ("Main Dashboard Buttons")
            (unwired) T25."Report" ("Main Dashboard Buttons")
            n795 = Not(x=w1048) -> (.not. x?=w1047:bool)
            n796 = local write "Zoom Factore"(0.0 ("Zoom Factore")) -> ()
            n797 = local write "Cap Live Image"(w1047) -> ()
            n798 = local write "Main Tab"(T2."Adv Scar Report" ("Main Tab")) -> ()
            n799 = property on="Cap Live Image" class="Bool (strict)"("BoolText.Text"="Capture Image" ("Boolean Text.Text")) -> ()  [unwired: 2 in, 2 out]
            n800 = local write "Main Dashboard Buttons"(T1."Report" ("Main Dashboard Buttons")) -> ()
          }
        }
      }
    }
    n801 = local read "change Gain"() -> (w694:bool)
    n802 = local read "Back Square"() -> (w693:bool)
    n803 = case shown="True" w694 {
      selector: w694 -> [_ w738]
      frame False {
      }
      frame True {
        n804 = stacked-sequence {
          tunnel: w738 -> [_ w746]
          frame #0 {
            n805 = local read "Actual (µm)"() -> (w742:dbl)
            n806 = local read "Pixel Value"() -> (w741:dbl)
            n807 = local read "Magnification :"() -> (w740:string)
            n808 = Divide(x=w742, y=w741) -> (x/y=w739:dbl)
            n809 = case shown="\"10x\"" w740 {
              tunnel: w739 -> [w743 w744]
              frame "10x" {
                n810 = local write "10x Gain"(w743) -> ()
              }
              frame "5x", Default {
                n811 = local write "5x Gain"(w744) -> ()
              }
            }
          }
          frame #1 {
            n812 = Not(x=w746) -> (.not. x?=w745:bool)
            n813 = local write "change Gain"(w745) -> ()
          }
        }
      }
    }
    n814 = case shown="True" w693 {
      selector: w693 -> [_ w736]
      frame False {
      }
      frame True {
        n815 = Not(x=w736) -> (.not. x?=w735:bool)
        n816 = local write "Back Square"(w735) -> ()
        n817 = local write "Calibration Tab"(enum32{"Measrument", "Calibrate"}."Measrument" ("Calibration Tab")) -> ()
      }
    }
    n818 = local read "Rectangle Tool"() -> (w705:bool)
    n819 = local read "Clear ROI Tool"() -> (w704:bool)
    n820 = local read "Open Image"() -> (w709:bool)
    n821 = local read "line tool"() -> (w706:bool)
    n822 = local read "OUT"() -> (w707:bool)
    n823 = local read "In"() -> (w708:bool)
    n824 = case shown="True" w709 {
      selector: w709 -> [_ w1014]
      tunnel: [w1010 w1016] -> _
      tunnel: w699 -> [w1010 w1015]
      frame False {
      }
      frame True {
        n825 = Not(x=w1014) -> (.not. x?=w1013:bool)
        n826 = local write "Open Image"(w1013) -> ()
        n827 = call "IMAGE ANALYSIS.vi"("Enum"=POST_ANALYSIS_ENUM."HIDE UI", "error in"=w1015) -> ("error out"=w1023:errorcluster)  [unwired: 8 in, 1 out]
        n828 = call "File Dialog"("start path"=path "C:/LAB-IQ/images", "error in"=w1023) -> ("selected path"=w1012:path, "error out"=w1021:errorcluster)  [unwired: 10 in, 2 out]
        "Image path  2" <- w1012
        n829 = call <vilib>:"Clear Errors.vi"("error in (no error)"=w1021) -> ("error out"=w1020:errorcluster)  [unwired: 5 in, 1 out]
        n830 = call "IMAGE ANALYSIS.vi"("Enum"=POST_ANALYSIS_ENUM."OPEN FILE", "error in"=w1020, "File Path"=w1012) -> ("error out"=w1019:errorcluster)  [unwired: 7 in, 1 out]
        n831 = call <vilib>:"Clear Errors.vi"("error in (no error)"=w1019) -> ("error out"=w1018:errorcluster)  [unwired: 5 in, 1 out]
        n832 = call "IMAGE ANALYSIS.vi"("Enum"=POST_ANALYSIS_ENUM."SHOW UI", "error in"=w1018) -> ("error out"=w1016:errorcluster)  [unwired: 8 in, 1 out]
        n833 = local write "Zoom Factore"(100.0 ("Zoom Factore")) -> ()
      }
    }
    n834 = case shown="True" w707 {
      selector: w707 -> [_ w995]
      tunnel: w699 -> [w992 w1000]
      tunnel: [w992 w994] -> _
      frame False {
      }
      frame True {
        n835 = Not(x=w995) -> (.not. x?=w993:bool)
        n836 = local read "Zoom Factore"() -> (w998:dbl)
        n837 = local write "OUT"(w993) -> ()
        n838 = call "IMAGE ANALYSIS.vi"("Enum"=POST_ANALYSIS_ENUM."ZOOM OUT", "error in"=w1000) -> ("error out"=w994:errorcluster)  [unwired: 8 in, 1 out]
        n839 = Divide(x=w998, y=1.2) -> (x/y=w996:dbl)
        n840 = local write "Zoom Factore"(w996) -> ()
      }
    }
    n841 = case shown="True" w708 {
      selector: w708 -> [_ w1004]
      tunnel: w699 -> [w1001 w1009]
      tunnel: [w1001 w1002] -> _
      frame False {
      }
      frame True {
        n842 = Not(x=w1004) -> (.not. x?=w1003:bool)
        n843 = local read "Zoom Factore"() -> (w1007:dbl)
        n844 = local write "In"(w1003) -> ()
        n845 = call "IMAGE ANALYSIS.vi"("Enum"=POST_ANALYSIS_ENUM."ZOOM IN", "error in"=w1009) -> ("error out"=w1002:errorcluster)  [unwired: 8 in, 1 out]
        n846 = Multiply(x=w1007, y=1.2) -> (x*y=w1005:dbl)
        n847 = local write "Zoom Factore"(w1005) -> ()
      }
    }
    n848 = case shown="True" w704 {
      selector: w704 -> [_ w976]
      tunnel: w699 -> [w974 w978]
      tunnel: [w974 w977] -> _
      frame False {
      }
      frame True {
        n849 = Not(x=w976) -> (.not. x?=w975:bool)
        n850 = local write "Clear ROI Tool"(w975) -> ()
        n851 = call "IMAGE ANALYSIS.vi"("Enum"=POST_ANALYSIS_ENUM."CLEAR ROI", "error in"=w978) -> ("error out"=w977:errorcluster)  [unwired: 8 in, 1 out]
      }
    }
    n852 = case shown="True" w706 {
      selector: w706 -> [_ w988]
      tunnel: w699 -> [w986 w991]
      tunnel: [w986 w989] -> _
      frame False {
      }
      frame True {
        n853 = Not(x=w988) -> (.not. x?=w987:bool)
        n854 = local write "line tool"(w987) -> ()
        n855 = call "IMAGE ANALYSIS.vi"("Enum"=POST_ANALYSIS_ENUM."DRAW LINE", "error in"=w991) -> ("error out"=w989:errorcluster)  [unwired: 8 in, 1 out]
      }
    }
    n856 = case shown="True" w705 {
      selector: w705 -> [_ w982]
      tunnel: w699 -> [w980 w984]
      tunnel: [w980 w983] -> _
      frame False {
      }
      frame True {
        n857 = Not(x=w982) -> (.not. x?=w981:bool)
        n858 = local write "Rectangle Tool"(w981) -> ()
        n859 = call "IMAGE ANALYSIS.vi"("Enum"=POST_ANALYSIS_ENUM."DRAW REC", "error in"=w984) -> ("error out"=w983:errorcluster)  [unwired: 8 in, 1 out]
      }
    }
    n860 = local read "SCAR MEASURMENT"() -> (w692:enum32{"Auto Scar", "Manual Scar"})
    n861 = local read "Fit to Screen Tool"() -> (w701:bool)
    n862 = local read "Resize Tool"() -> (w700:bool)
    n863 = case shown="\"Manual Scar\", Default" w692 {
      frame "Auto Scar" {
        n864 = property on="Cap Live Image" class="Bool (strict)"("BoolText.Text"="Report" ("Boolean Text.Text")) -> ()  [unwired: 2 in, 2 out]
      }
      frame "Manual Scar", Default {
        n865 = property on="Cap Live Image" class="Bool (strict)"("BoolText.Text"="Save Image" ("Boolean Text.Text")) -> ()  [unwired: 2 in, 2 out]
      }
    }
    n866 = local read "ROI Color Tool"() -> (w702:bool)
    n867 = local read "Pan Tool"() -> (w703:bool)
    n868 = case shown="True" w703 {
      selector: w703 -> [_ w970]
      tunnel: w699 -> [w968 w972]
      tunnel: [w968 w971] -> _
      frame False {
      }
      frame True {
        n869 = Not(x=w970) -> (.not. x?=w969:bool)
        n870 = call "IMAGE ANALYSIS.vi"("Enum"=POST_ANALYSIS_ENUM."PAN", "error in"=w972) -> ("error out"=w971:errorcluster)  [unwired: 8 in, 1 out]
        n871 = local write "Pan Tool"(w969) -> ()
      }
    }
    n872 = case shown="True" w700 {
      selector: w700 -> [_ w954]
      tunnel: w699 -> [w949 w951]
      tunnel: [w949 w950] -> _
      frame False {
      }
      frame True {
        n873 = Not(x=w954) -> (.not. x?=w953:bool)
        n874 = local write "Resize Tool"(w953) -> ()
        n875 = call "IMAGE ANALYSIS.vi"("Enum"=POST_ANALYSIS_ENUM."RESIZE MODE", "error in"=w951) -> ("error out"=w950:errorcluster)  [unwired: 8 in, 1 out]
      }
    }
    n876 = case shown="True" w701 {
      selector: w701 -> [_ w959]
      tunnel: [w955 w960] -> _
      tunnel: w699 -> [w955 w958]
      frame False {
      }
      frame True {
        n877 = Not(x=w959) -> (.not. x?=w957:bool)
        n878 = local write "Zoom Factore"(100.0 ("Zoom Factore")) -> ()
        n879 = local write "Fit to Screen Tool"(w957) -> ()
        n880 = call "IMAGE ANALYSIS.vi"("Enum"=POST_ANALYSIS_ENUM."FIT", "error in"=w958) -> ("error out"=w960:errorcluster)  [unwired: 8 in, 1 out]
      }
    }
    n881 = case shown="True" w702 {
      selector: w702 -> [_ w965]
      tunnel: [w962 w966] -> _
      tunnel: w699 -> [w962 w963]
      frame False {
      }
      frame True {
        n882 = Not(x=w965) -> (.not. x?=w964:bool)
        n883 = local write "ROI Color Tool"(w964) -> ()
        n884 = call "IMAGE ANALYSIS.vi"("Enum"=POST_ANALYSIS_ENUM."SET ROI COLOR", "error in"=w963) -> ("error out"=w966:errorcluster)  [unwired: 8 in, 1 out]
      }
    }
    n885 = local read "Quit"() -> (w716:bool)
  }
  n886 = while {
    stop <- w1050 stop-if-true
    n887 = local read "Image Path"() -> (w1053:path)
    n888 = local read "Print 3"() -> (w1056:bool)
    n889 = Equal?(x=w1053, y=path "") -> (x = y?=w1052:bool)
    n890 = Not(x=w1052) -> (.not. x?=w1051:bool)
    n891 = property on="Print 3" class="Bool (strict)"("Visible"=w1051) -> ()  [unwired: 2 in, 2 out]
    n892 = case shown="True" w1056 {
      frame False {
        n893 = local write "Rd"(TRUE ("Boolean 7")) -> ()
      }
      frame True {
        n894 = flat-sequence {
          tunnel: [w1096] -> w1064
          tunnel: [w1083] -> w1062
          tunnel: [w1093] -> w1058
          tunnel: w1064 -> [w1105]
          tunnel: [w1105] -> w1063
          tunnel: w1062 -> [w1104]
          tunnel: [w1104] -> w1061
          tunnel: [w1102] -> w1060
          tunnel: [w1101] -> w1059
          tunnel: w1058 -> [w1101]
          tunnel: w1063 -> [w1107]
          tunnel: w1061 -> [w1108]
          tunnel: w1060 -> [_]
          tunnel: w1059 -> [w1106]
          frame #0 {
            n895 = case shown="True" "Rd" {
              frame False {
              }
              frame True {
                n896 = while {
                  tunnel: "abcdefABCDEF" ("string 2") -> [w1075]
                  shift-right: [w1073] -> w1067
                  shift-left: "" -> [w1072]
                  i -> [w1082]
                  stop <- w1081 stop-if-true
                  n897 = Random Number (0-1)() -> (number: 0 to 1=w1076:dbl)
                  n898 = Multiply(x=w1076, y=62.0) -> (x*y=w1078:dbl)
                  n899 = Decrement(x="Length 2") -> (x-1=w1071:i16)
                  n900 = To Word Integer(number=w1078) -> (16bit integer=w1079:i16)
                  n901 = String Subset(string=w1075, offset (0)=w1079, length (rest)=1 ("length (rest)")) -> (substring=w1074:string)
                  n902 = Greater Or Equal?(x=w1082, y=w1071) -> (x >= y?=w1081:bool)
                  n903 = Concatenate Strings(w1074, w1072) -> (w1073:string)
                }
                "String 10" <- w1067
                n904 = local write "Rd"(FALSE ("Boolean 7")) -> ()
              }
            }
          }
          frame #1 {
            w1094 = "_resized.jpg" ("command line")
            (unwired) ".jpg -resize 320x240 " ("string")
            (unwired) "Choose an Image File" ("prompt")
            # "-resize 1798x425"
            n905 = local read "Image Path"() -> (w1088:path)
            n906 = Strip Path(path=w1088) -> (stripped path=w1083:path, name=w1084:string)
            n907 = Match Pattern(string=w1084, regular expression=".jpg") -> (before substring=→"before substring 2":string, after substring=→"after substring":string)  [unwired: 1 in, 2 out]
            n908 = Match Pattern(string=w1084, regular expression="\\") -> (before substring=w1090:string)  [unwired: 1 in, 3 out]
            n909 = Match Pattern(string=w1090, regular expression=".jpg") -> (before substring=w1089:string)  [unwired: 1 in, 3 out]
            n910 = Concatenate Strings("cmd /c convert " ("string"), w1089, ".jpg -resize 320x240  " ("command line"), w1089, w1094) -> (w1097:string)
            n911 = call <vilib>:"System Exec.vi"("run minimized? (F)"=TRUE, "wait until completion? (T)"=TRUE, "working directory"=w1083, "command line"=w1097) -> ("error out"=w1096:errorcluster)  [unwired: 4 in, 3 out]
            "error out 2" <- w1096
            n912 = Concatenate Strings(w1089, w1094) -> (w1093:string)
          }
          frame #2 {
            n913 = Wait (ms)(milliseconds to wait=u32 2000 ("millisecond timer value")) -> (millisecond timer value=w1102:u32)
          }
          frame #3 {
            n914 = case shown="No Error" w1107 {
              tunnel: w1108 -> [w1111 _]
              tunnel: w1106 -> [w1109 _]
              frame No Error {
                (unwired) ".jpg" ("string")
                n915 = Path To String(path=w1111) -> (string=w1115:string)
                n916 = Concatenate Strings(w1115, "\\" ("string"), w1109) -> (w1114:string)
                n917 = String To Path(string=w1114) -> (path=w1113:path)
                n918 = call <vilib>:"Read JPEG File.vi"("path to JPEG file"=w1113) -> ("image data"=w1117:T15)  [unwired: 8 in, 2 out]
                "image data" <- w1117
                n919 = local write "Print 3"(FALSE ("Print 2")) -> ()
                n920 = call <vilib>:"Draw Flattened Pixmap.vi"("image data"=w1117) -> ("new picture"=→"new picture":picture)  [unwired: 8 in]
              }
              frame Error {
              }
            }
          }
        }
      }
    }
